vi "cg_Line Minimum Fletcher.vi"(6 "zeps":dbl=1e-12 format="%.2e", 7 "function and data":T1, 8 "error in (no error)":errorcluster, 9 "tol":dbl=1e-06 format="%.2e", 10 "p":dbl[](array[numeric]) format="%.2f", 11 "xit":dbl[](array[numeric]) format="%.2f") -> (0 "error out":errorcluster, 1 "f(p)":dbl format="%.2f", 2 "pnew":dbl[](array[numeric]) format="%.2f", 3 "xitnew":dbl[](array[numeric]) format="%.2f", 5 "number of function calls":i32)   [LabVIEW 2010, in "NI_Gmath.lvlib"]
uses:
  NI_Gmath.lvlib
  ucno_user function ref and data.ctl
  ucno_user objective function ref.ctl
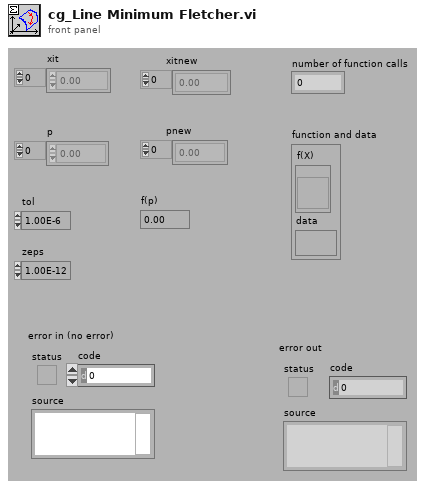
[diagram p1: front panel]
types:
  T1 = typedef "NI_Gmath.lvlib/ucno_user function ref and data.ctl" = cluster{"f(X)":T2, "data":variant}
  T2 = typedef "NI_Gmath.lvlib/ucno_user objective function ref.ctl" = refnum<vi>
  T3 = cluster{"objective function":bool, "gradient":bool}
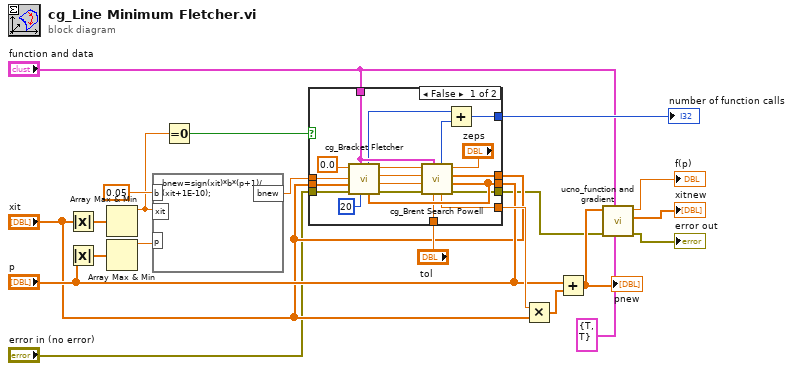
[diagram p0: block diagram]
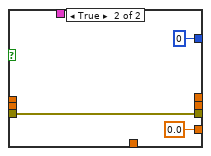
[diagram p2: hidden frame]
diagram:
  n1 = Absolute Value(x="xit") -> (abs(x)=w13:dbl[])
  n2 = Absolute Value(x="p") -> (abs(x)=w12:dbl[])
  n3 = Array Max & Min(array=w13) -> (max value=w8:dbl)  [unwired: 3 out]
  n4 = Array Max & Min(array=w12) -> (max value=w11:dbl)  [unwired: 3 out]
  n5 = formula code="bnew=sign(xit)*b*(p+1)/(xit+1E-10);"("b"=0.05, "xit"=w8, "p"=w11) -> ("bnew"=w9:dbl)
  n6 = Equal To 0?(x=w8) -> (x = 0?=w6:bool)
  n7 = case shown="False" w6 {
    tunnel: w9 -> [w38 _]
    tunnel: "xit" -> [w30 _]
    tunnel: "p" -> [w37 _]
    tunnel: [w36 0.0] -> w19
    tunnel: "tol" -> [w34 _]
    tunnel: "xit" -> [w29 _]
    tunnel: "function and data" -> [w26 _]
    tunnel: "error in (no error)" -> [w28 w42]
    tunnel: [w25 w42] -> w3
    tunnel: [w22 0] -> w21
    frame False {
      n8 = call "cg_Bracket Fletcher.vi"("p"=w37, "loops"=u32 20, "function and data"=w26, "error in (no error)"=w28, "xit"=w29, "b (start)"=w38, "a (start)"=0.0) -> ("error out"=w27:errorcluster, "c (bracket)"=w33:dbl, "b (bracket)"=w32:dbl, "a (bracket)"=w31:dbl, "number of function calls"=w23:i32)
      n9 = call "cg_Brent Search Powell.vi"("p"=w37, "xit"=w30, "ZEPS"="zeps", "tol"=w34, "function and data"=w26, "error in (no error)"=w27, "c (start)"=w33, "b (start)"=w32, "a (start)"=w31) -> ("error out"=w25:errorcluster, "u"=w36:dbl, "number of function calls"=w24:i32)
      n10 = Add(x=w23, y=w24) -> (x+y=w22:i32)
    }
    frame True {
    }
  }
  "number of function calls" <- w21
  n11 = Multiply(x=w19, y="xit") -> (x*y=w16:dbl[])
  n12 = Add(x="p", y=w16) -> (x+y=w18:dbl[])
  "pnew" <- w18
  n13 = call "ucno_function and gradient.vi"("output control"=T3 {"objective function"=TRUE, "gradient"=TRUE}, "function and data"="function and data", "error in (no error)"=w3, "X"=w18) -> ("error out"=→"error out":errorcluster, "gradient"=→"xitnew":dbl[], "f(X)"=→"f(p)":dbl)  [unwired: 4 in, 1 out]
